vi "ControllerPersistor.vi"(1 "status":string, 2 "controller_id":string, 3 "controller parameters":cluster{"Kc":dbl, "Ti":dbl, "Td":dbl}={"Kc"=1.0, "Ti"=40.0, "Td"=0.0}, 4 "controller_output":dbl, 5 "controller_input":dbl, 6 "controller_setpoint":dbl) -> (0 "结果字符串":string)   [LabVIEW 2016]
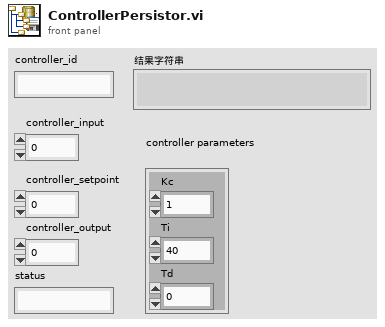
[diagram p1: front panel]
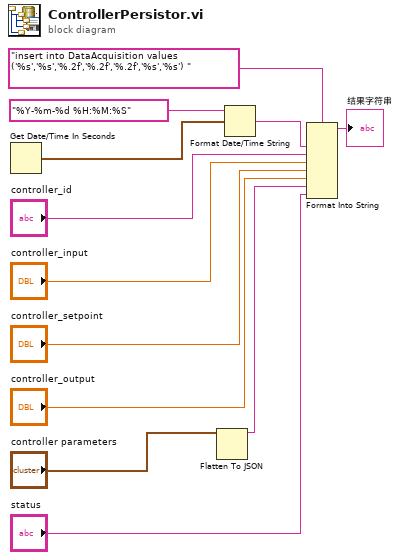
[diagram p0: block diagram]
diagram:
  n1 = Get Date/Time In Seconds() -> (seconds since 1Jan1904=w11:timestamp)
  n2 = Flatten To JSON(anything="controller parameters") -> (JSON string=w3:string)  [unwired: 2 in, 1 out]
  n3 = Format Date/Time String ("格式化日期/时间字符串")(time format string (%c)="%Y-%m-%d %H:%M:%S" ("时间格式字符串(%c)"), seconds (now)=w11) -> (date/time string=w9:string)  [unwired: 1 in]
  n4 = Format Into String(format string="insert into DataAcquisition values ('%s','%s','%.2f','%.2f','%.2f','%s','%s') " ("格式字符串"), w9, "controller_id", "controller_input", "controller_setpoint", "controller_output", w3, "status") -> (resulting string=→"结果字符串":string)  [unwired: 2 in, 1 out]
